vi "Pack State Sample Message.vi"(11 "State Sample":refnum<class "RDS State.lvclass">) -> (3 "State Sample Message out":refnum<class "State Sample Message.lvclass">)   [LabVIEW 2015, in "RDS State Tracker.lvlib"]
uses:
  RDS State Tracker.lvlib
  RDS State/RDS State.lvclass
  Libraries/RDS Child Messages/State Sample Message/State Sample Message.lvclass
  Libraries/RDS Framework/RDS Message ID.ctl
  Libraries/RDS Framework/RDS Message Class/RDS Message.lvclass/RDS Message.ctl
  Libraries/RDS Child Messages/State Sample Message/State Sample Message.lvclass/State Sample Message.ctl
  Libraries/RDS Framework/RDS Message Class/RDS Message.lvclass
  Libraries/RDS Child Messages/RDS Child Messages.lvlib
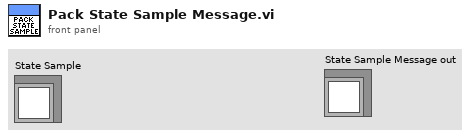
[diagram p1: front panel]
types:
  T1 = typedef "RDS Child Messages.lvlib/RDS Message ID.ctl" = enum16{"RDS Hello World", "String Message", "AIP_Status", "AIP_Command", "GPS_Data", "MCB_Command", "MCB_Status", "Compass_Data", "Depth_Data", "Battery_Data", "Contoller_State", "Set_Mag_Dev", "BTB_Shutdown", "State_Sample_Request", "State_Sample", "PID_Gains_Set", "Helm_Limiter_Set", "Helm_Heading_Command", "Helm_Steering_Command", "Helm_Status", "Controller_Message", "AIP_Set_Min_Depth", "Mission_Controller_State", "Mission_Upload", "Mission_Set_Op_and_Run", "Mission_Settings_Set"}
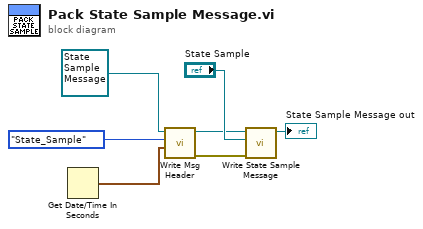
[diagram p0: block diagram]
diagram:
  n1 = Get Date/Time In Seconds() -> (seconds since 1Jan1904=w7:timestamp)
  n2 = call "Write Msg Header.vi"("Time Stamp"=w7, "Msg ID"=RDS_Message_ID."State_Sample", "RDS Message in"=refnum<class "State Sample Message.lvclass"> refnum ("RDS Child Messages.lvlib:State Sample Message.lvclass")) -> ("error out"=w2:errorcluster, "RDS Message out"=w3:refnum<class "State Sample Message.lvclass">)  [unwired: 7 in]
  n3 = call "Write State Sample Message.vi"("error in (no error)"=w2, "RDS State Tracker.lvlib:RDS State.lvclass"="State Sample", "State Sample Message in"=w3) -> ("State Sample Message out"=→"State Sample Message out":refnum<class "State Sample Message.lvclass">)  [unwired: 7 in, 1 out]
